vi "VisionNetwork.vi"(8 "error in (no error)":errorcluster) -> (0 "error out":errorcluster)   [LabVIEW 2020]
doc: "Vision Network\n\nInput\n --Error in \n\nOutput\n --Error out"
uses:
  <vilib>/Rock Robotics/WPI/ThirdParty/JAS_Junk/TrajLib/Trajectory_Library.lvlib
  <vilib>/Rock Robotics/Network Tables/NT Write Number.vi
  <vilib>/Rock Robotics/Network Tables/NT Write Boolean.vi
  <vilib>/Rock Robotics/Network Tables/NT Read Number.vi
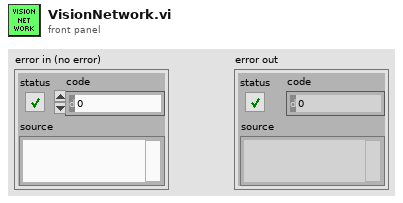
[diagram p1: front panel]
types:
  T1 = typedef "Trajectory_Library.lvlib/POSE2D.ctl" = cluster{"TRANSLATION":T2, "ROTATION":T3}
  T2 = typedef "Trajectory_Library.lvlib/TRANSLATION2D.ctl" = cluster{"X":dbl, "Y":dbl}
  T3 = typedef "Trajectory_Library.lvlib/ROTATION2D.ctl" = cluster{"VALUE":dbl, "COS":dbl, "SIN":dbl}
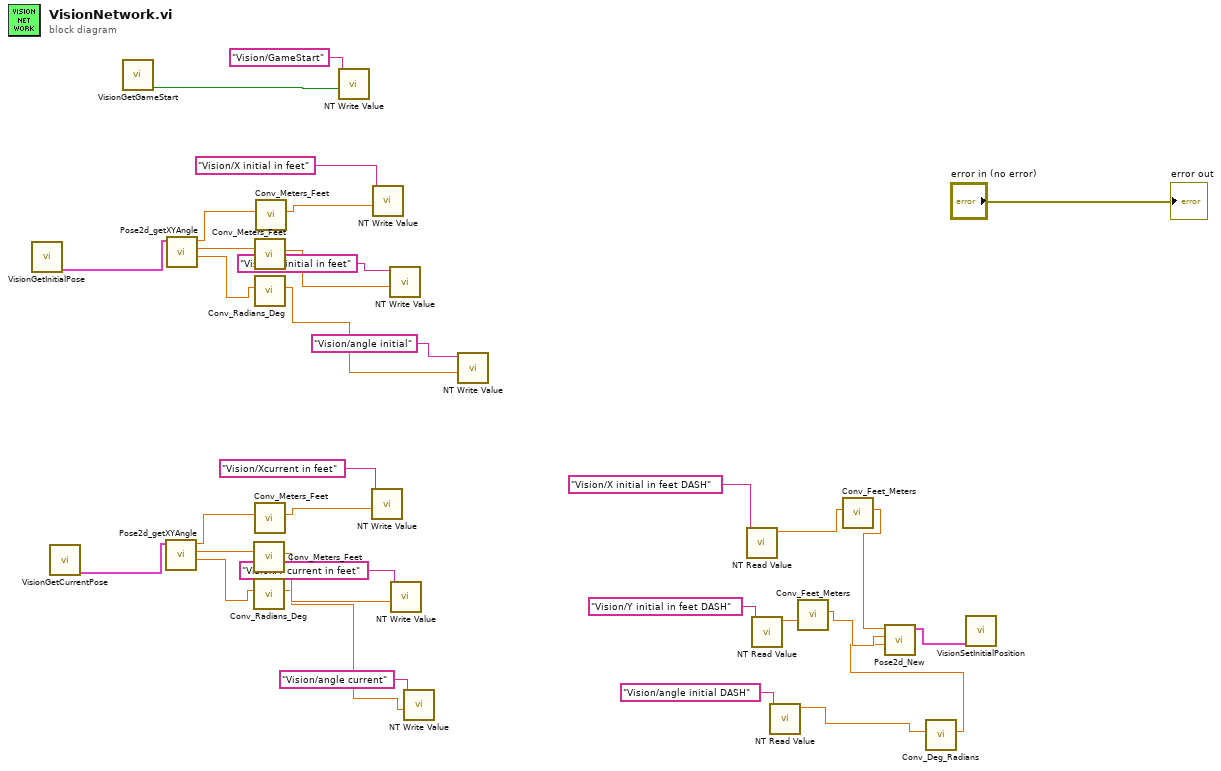
[diagram p0: block diagram]
diagram:
  n1 = call "VisionGetInitialPose.vi"() -> ("InitialPose"=w19:T1)  [unwired: 10 in]
  n2 = call "VisionGetCurrentPose.vi"() -> ("Current Pose"=w32:T1)  [unwired: 9 in]
  n3 = call "VisionGetGameStart.vi"() -> ("Game Start"=w18:bool)  [unwired: 11 in]
  n4 = call <vilib>:"Pose2d_getXYAngle.vi"("in POSE"=w32) -> ("Angle"=w31:dbl, "Y"=w30:dbl, "X"=w29:dbl)  [unwired: 8 in]
  n5 = call <vilib>:"Pose2d_getXYAngle.vi"("in POSE"=w19) -> ("Angle"=w25:dbl, "Y"=w24:dbl, "X"=w23:dbl)  [unwired: 8 in]
  n6 = call <vilib>:"Conv_Meters_Feet.vi"("Meters"=w30) -> ("Feet"=w27:dbl)  [unwired: 10 in]
  n7 = call <vilib>:"Conv_Radians_Deg.vi"("Radians"=w31) -> ("Degrees"=w26:dbl)  [unwired: 10 in]
  n8 = call <vilib>:"Conv_Meters_Feet.vi"("Meters"=w24) -> ("Feet"=w21:dbl)  [unwired: 10 in]
  n9 = call <vilib>:"Conv_Radians_Deg.vi"("Radians"=w25) -> ("Degrees"=w20:dbl)  [unwired: 10 in]
  n10 = call <vilib>:"Conv_Meters_Feet.vi"("Meters"=w29) -> ("Feet"=w28:dbl)  [unwired: 10 in]
  n11 = call <vilib>:"Conv_Meters_Feet.vi"("Meters"=w23) -> ("Feet"=w22:dbl)  [unwired: 10 in]
  n12 = call-poly <vilib>:"NT Write Value.vi"("value"=w18, "name"="Vision/GameStart") -> ()  [unwired: 9 in, 1 out]
  n13 = call-poly <vilib>:"NT Write Value.vi"("value"=w28, "name"="Vision/Xcurrent in feet") -> ()  [unwired: 9 in, 1 out]
  n14 = call-poly <vilib>:"NT Write Value.vi"("value"=w22, "name"="Vision/X initial in feet") -> ()  [unwired: 9 in, 1 out]
  n15 = call-poly <vilib>:"NT Write Value.vi"("value"=w21, "name"="Vision/Y initial in feet") -> ()  [unwired: 9 in, 1 out]
  n16 = call-poly <vilib>:"NT Write Value.vi"("value"=w27, "name"="Vision/Y current in feet") -> ()  [unwired: 9 in, 1 out]
  n17 = call-poly <vilib>:"NT Write Value.vi"("value"=w26, "name"="Vision/angle current") -> ()  [unwired: 9 in, 1 out]
  n18 = call-poly <vilib>:"NT Write Value.vi"("value"=w20, "name"="Vision/angle initial") -> ()  [unwired: 9 in, 1 out]
  n19 = call-poly <vilib>:"NT Read Value.vi"("name"="Vision/X initial in feet DASH") -> ("value"=w8:dbl)  [unwired: 8 in, 2 out]
  n20 = call-poly <vilib>:"NT Read Value.vi"("name"="Vision/Y initial in feet DASH") -> ("value"=w7:dbl)  [unwired: 8 in, 2 out]
  n21 = call-poly <vilib>:"NT Read Value.vi"("name"="Vision/angle initial DASH") -> ("value"=w5:dbl)  [unwired: 8 in, 2 out]
  n22 = call <vilib>:"Conv_Feet_Meters.vi"("Feet"=w7) -> ("Meters"=w6:dbl)  [unwired: 10 in]
  n23 = call <vilib>:"Conv_Feet_Meters.vi"("Feet"=w8) -> ("Meters"=w9:dbl)  [unwired: 10 in]
  n24 = call <vilib>:"Conv_Deg_Radians.vi"("Degress"=w5) -> ("Radians"=w4:dbl)  [unwired: 10 in]
  n25 = call <vilib>:"Pose2d_New.vi"("Heading"=w4, "Y"=w6, "X"=w9) -> ("out POSe"=w10:T1)  [unwired: 8 in]
  n26 = call "VisionSetInitialPosition.vi"("InitialPose"=w10) -> ()  [unwired: 11 in]
  "error out" <- "error in (no error)"
